vi "SENS_CORR_COLL_GUID_SAVE.vi"(0 "VISA IN":refnum<visa-resource-name>, 1 "Calset":string, 5 "error in":errorcluster, 7 "Channel":i32) -> (14 "VISA Out":refnum<visa-resource-name>, 19 "error out":errorcluster)   [LabVIEW 2018, in "PNA-X.lvlib"]
doc: "SENSe:CORRection:COLLect:GUIDed:SAVE:CSET <cal set name or guid>\n(Write-only) Completes the guided cal by computing the error correction terms, turning Correction ON, and saving the calibration to the specified Cal Set. This command performs the same function as SENSe:CORRection:COLLect:GUIDed:SAVE, but this command allows the name or GUID of the Cal Set to be specified.\n\nUse this command instead of the optional name or GUID argument in SENS:CORR:COLL:GUID:INIT.\n\nUse SENS:CORRection:CSET commands to get names or GUIDs of existing Cal Sets.\n\nThe cal data is also saved to the channel Cal Register.\n\nIf all of the required standards have not been measured, the calibration will not complete properly.\n \nParameters\n \n \n<cal set name or guid>\n String - Name or GUID of an existing Cal Set to be overwritten. If specifying a GUID, curly brackets must be included.\n \nExamples\n SENS:CORR:COLL:GUID:SAVE:CSET \"{2B893E7A-971A-11d5-8D6C-00108334AE96}\"\n\nsense:correction:collect:guided:save:cset \"MyCalSet\"\n \nQuery Syntax\n Not Applicable\n \nDefault\n Not Applicable"
uses:
  PNA-X.lvlib
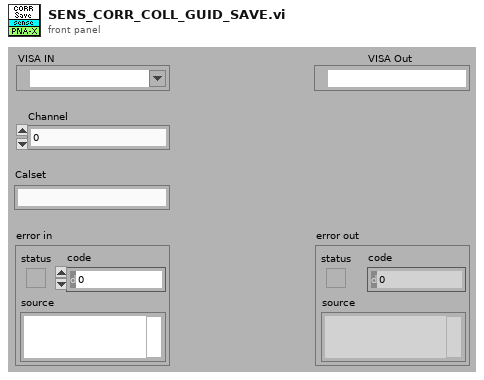
[diagram p1: front panel]
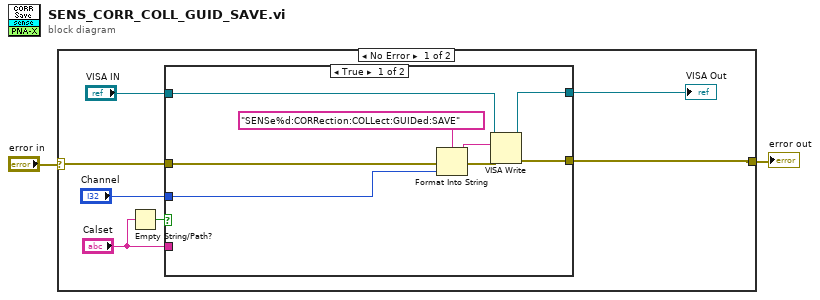
[diagram p0: block diagram]
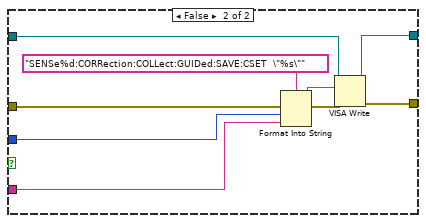
[diagram p2: hidden frame]
diagram:
  n1 = case shown="No Error" "error in" {
    selector: "error in" -> [w9 w27]
    tunnel: [w7 w27] -> w1
    frame No Error {
      n2 = Empty String/Path?(string/path="Calset") -> (empty?=w3:bool)
      n3 = case shown="True" w3 {
        tunnel: w9 -> [w17 w26]
        tunnel: "VISA IN" -> [w14 w23]
        tunnel: [w12 w21] -> w7
        tunnel: [w11 w20] -> w6
        tunnel: "Channel" -> [w10 w19]
        tunnel: "Calset" -> [_ w18]
        frame True {
          n4 = Format Into String(format string="SENSe%d:CORRection:COLLect:GUIDed:SAVE" ("Cmdline"), error in=w17, w10) -> (resulting string=w15:string, error out=w16:errorcluster)  [unwired: 1 in]
          n5 = VISA Write(VISA resource name=w14, write buffer=w15, error in (no error)=w16) -> (VISA resource name out=w11:refnum<visa-resource-name>, error out=w12:errorcluster)  [unwired: 1 out]
        }
        frame False {
          n6 = Format Into String(format string="SENSe%d:CORRection:COLLect:GUIDed:SAVE:CSET  \"%s\"" ("Cmdline"), error in=w26, w19, w18) -> (resulting string=w24:string, error out=w25:errorcluster)  [unwired: 1 in]
          n7 = VISA Write(VISA resource name=w23, write buffer=w24, error in (no error)=w25) -> (VISA resource name out=w20:refnum<visa-resource-name>, error out=w21:errorcluster)  [unwired: 1 out]
        }
      }
      "VISA Out" <- w6
    }
    frame Error {
    }
  }
  "error out" <- w1
